vi "Read Time Entry.vi"(8 "error in (no error)":errorcluster, 10 "GUID":string, 11 "Time Entry-INI in":refnum<class "Time Entry-INI.lvclass">) -> (0 "error out":errorcluster, 3 "Time Entry-INI out":refnum<class "Time Entry-INI.lvclass">)   [LabVIEW 2020, in "Time Entry-INI.lvclass"]
doc: "VI for override that will read the specific time entry from the file/database/other specified for record keeping. The GUID is used because that is a unique way of identifying an entry.\n\n04/2025 Erich Schlieper"
uses:
  Time Entry-INI.lvclass
  C:/Apps/LVTimeTracker/LVTimeTracker/Time Entries/Time Entry/Time Entries.lvclass
  Time Entry-INI.lvclass/Time Entry-INI.ctl
  <vilib>/Utility/config.llb/Read Key (String).vi
  <vilib>/Utility/config.llb/Read Key (Double).vi
  Time Entry/Time Entries.lvclass
  <vilib>/Utility/config.llb/NI_LVConfig.lvlib
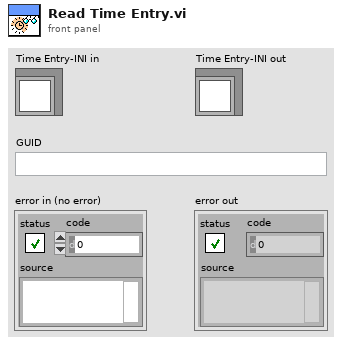
[diagram p1: front panel]
types:
  T1 = typedef "NI_LVConfig.lvlib/Config Data RefNum.ctl" = refnum<k1>
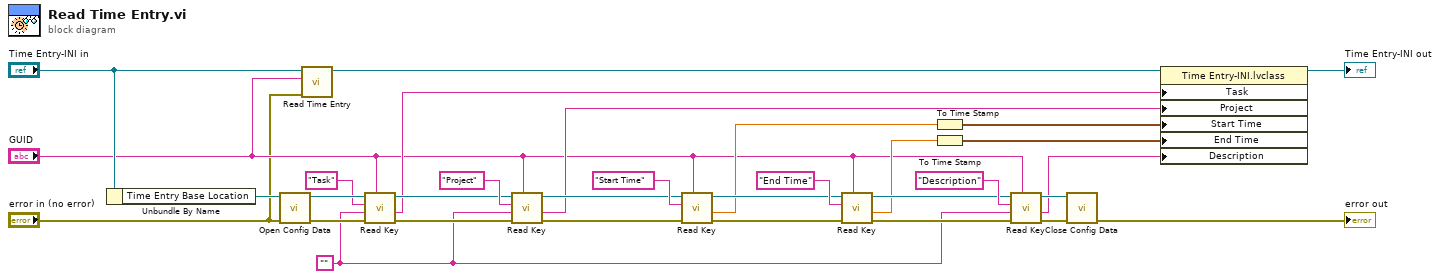
[diagram p0: block diagram]
diagram:
  w13 = ""
  n1 = Unbundle By Name("Time Entry-INI in") -> ("Time Entry Base Location"=w15:path)
  n2 = call <vilib>:"Open Config Data.vi"("error in (no error)"="error in (no error)", "configuration file path"=w15) -> ("error out"=w30:errorcluster, "refnum"=w32:T1)  [unwired: 7 in, 1 out]
  n3 = call-parent "Read Time Entry.vi"("error in (no error)"="error in (no error)", "GUID"="GUID", "Time Entries in"="Time Entry-INI in") -> ("Time Entries out"=w3:refnum<class "Time Entry-INI.lvclass">)  [unwired: 7 in, 1 out]
  n4 = call-poly <vilib>:"Read Key.vi"("section"="GUID", "error in (no error)"=w30, "default value"=w13, "key"="Task", "refnum"=w32) -> ("error out"=w21:errorcluster, "value"=w6:string, "refnum out"=w25:T1)  [unwired: 3 in, 1 out]
  n5 = call-poly <vilib>:"Read Key.vi"("section"="GUID", "error in (no error)"=w21, "default value"=w13, "key"="Project", "refnum"=w25) -> ("error out"=w20:errorcluster, "value"=w7:string, "refnum out"=w24:T1)  [unwired: 3 in, 1 out]
  n6 = call-poly <vilib>:"Read Key.vi"("section"="GUID", "error in (no error)"=w20, "key"="Start Time", "refnum"=w24) -> ("error out"=w19:errorcluster, "value"=w8:dbl, "refnum out"=w23:T1)  [unwired: 4 in, 1 out]
  n7 = call-poly <vilib>:"Read Key.vi"("section"="GUID", "error in (no error)"=w19, "key"="End Time", "refnum"=w23) -> ("error out"=w18:errorcluster, "value"=w9:dbl, "refnum out"=w22:T1)  [unwired: 4 in, 1 out]
  n8 = To Time Stamp(1:w8) -> (0:w10:timestamp)
  n9 = To Time Stamp(1:w9) -> (0:w11:timestamp)
  n10 = call-poly <vilib>:"Read Key.vi"("section"="GUID", "error in (no error)"=w18, "default value"=w13, "key"="Description", "refnum"=w22) -> ("error out"=w17:errorcluster, "value"=w12:string, "refnum out"=w16:T1)  [unwired: 3 in, 1 out]
  n11 = call <vilib>:"Close Config Data.vi"("error in (no error)"=w17, "refnum"=w16) -> ("error out"=→"error out":errorcluster)  [unwired: 8 in, 1 out]
  n12 = property class="Time Entry-INI.lvclass"(reference=w3, "Task"=w6, "Project"=w7, "Start Time"=w10, "End Time"=w11, "Description"=w12) -> (reference out=→"Time Entry-INI out":refnum<class "Time Entry-INI.lvclass">)  [unwired: 1 in, 1 out]
